vi "motor run.vi"(3 "Motor.brake":bool, 4 "dt(s)":dbl, 6 "motor select":T2, 7 "PID gains":T1={"proportional gain (Kc)"=1.0, "integral time (Ti, min)"=0.01, "derivative time (Td, min)"=0.0} {"derivative time (Td, min)" format="%.3f"; "integral time (Ti, min)" format="%.3f"; "proportional gain (Kc)" format="%.3f"}, 8 "error in":errorcluster, 9 "Reset":bool, 10 "speed RPM":dbl, 11 "PWM frequence":dbl=1250.0) -> (0 "error out":errorcluster, 1 "output":dbl format="%.2f", 2 "encoder":dbl, 5 "setpoint":dbl)   [LabVIEW 2019, in "my FPGA lib.lvlib" / "motor.lvlib"]
uses:
  motor.lvlib
  motor enum.ctl
  <vilib>/addons/control/pid/pid.llb/PID (DBL).vi
  my FPGA lib.lvlib
  <vilib>/addons/control/pid/NI_PID_pid.lvlib
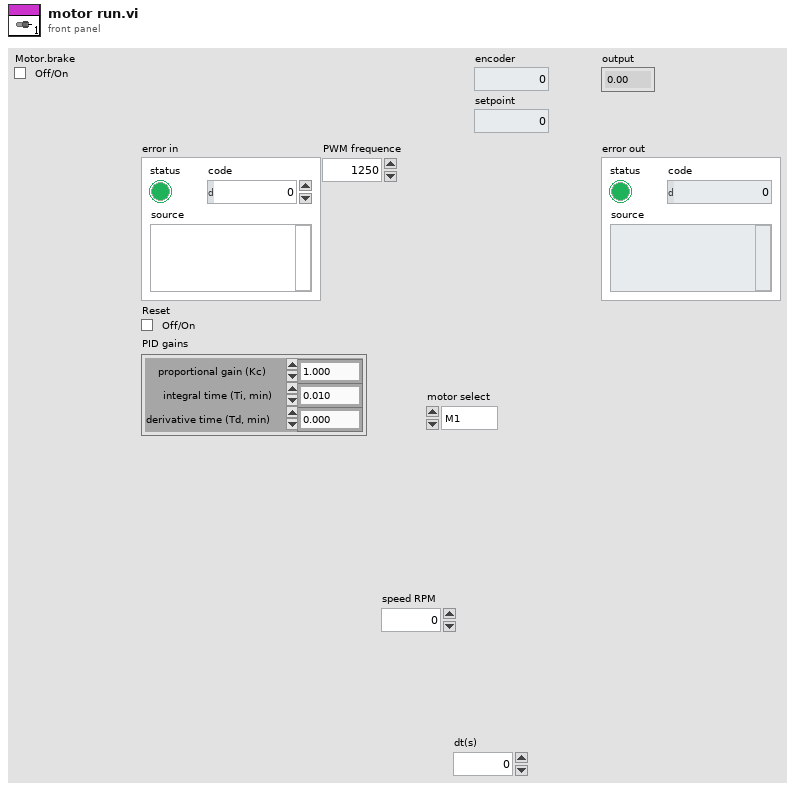
[diagram p1: front panel]
types:
  T1 = cluster{"proportional gain (Kc)":dbl, "integral time (Ti, min)":dbl, "derivative time (Td, min)":dbl}
  T2 = typedef "my FPGA lib.lvlib/motor.lvlib/motor enum.ctl" = enum16{"M1", "M2", "M3", "M4"}
  T3 = cluster{"divider rate":i32, "enable divider":bool, "period":i32}
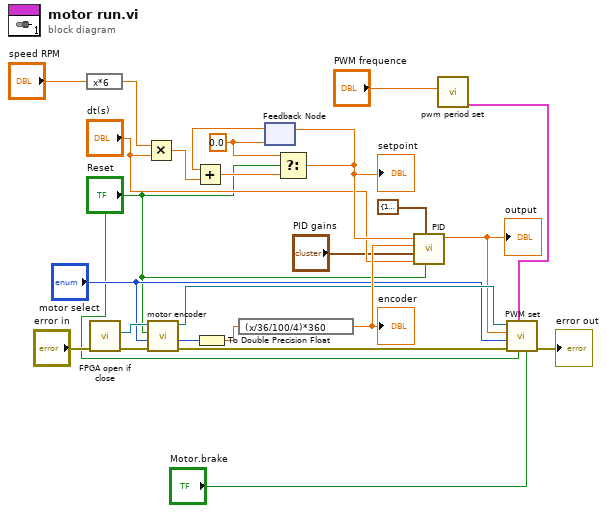
[diagram p0: block diagram]
diagram:
  w16 = 0.0 ("t")
  n1 = expression code="x*6"("speed RPM") -> (w19:dbl)
  n2 = call "FPGA open if close.vi"("error in"="error in") -> ("error out"=w24:errorcluster, "FPGA VI Reference Out"=w23:refnum<k20>)  [unwired: 9 in]
  n3 = Multiply(x=w19, y="dt(s)") -> (x*y=w15:dbl)
  n4 = call "motor encoder.vi"("Error In"=w24, "motor select"="motor select", "Reset"="Reset", "FPGA VI Reference In"=w23) -> ("error out"=w7:errorcluster, "encoder"=w22:i32, "FPGA VI Reference Out"=w8:refnum<k20>)  [unwired: 5 in]
  n5 = To Double Precision Float(number=w22) -> (double precision float=w21:dbl)
  n6 = expression code="(x/36/100/4)*360"(w21) -> (w13:dbl)
  "encoder" <- w13
  n7 = feedback #1(w16) -> (w17:dbl)
  n8 = Add(x=w17, y=w15) -> (x+y=w18:dbl)
  n9 = Select(t=w16, s="Reset", f=w18) -> (s? t:f=w14:dbl)
  "setpoint" <- w14
  n10 = feedback-in #1(w14) -> ()
  n11 = call-poly <vilib>:"PID.vi"("reinitialize? (F)"="Reset", "output range"=cluster{"output high":dbl, "output low":dbl} {"output high"=100.0, "output low"=-100.0}, "dt (s)"="dt(s)", "PID gains"="PID gains", "process variable"=w13, "setpoint"=w14) -> ("output"=w6:dbl)  [unwired: 4 in, 1 out]
  "output" <- w6
  n12 = call "pwm period set.vi"("PWM frequence"="PWM frequence") -> ("pwm cnfg"=w4:T3)  [unwired: 10 in]
  n13 = call "PWM set.vi"("Motor.brake"="Motor.brake", "Reset"="Reset", "pwm cnfg"=w4, "Error In"=w7, "motor select"="motor select", "PWM"=w6, "FPGA VI Reference In"=w8) -> ("error out"=→"error out":errorcluster)  [unwired: 4 in]
